vi "A33ConfigureFM.vi"(0 "VISA resource name":refnum<visa-resource-name>, 1 "Enable Frequency Modulation (T:Enable)":bool=TRUE, 2 "Modulation Frequency (1000.0 Hz)":dbl=1000.0 format="%#_12g", 5 "Channel (1: Channel1)":u16(ring)=1 items=["Channel1"=1, "Channel2"=2], 7 "FM Source (0: Internal)":u16(ring) items=["Internal", "External", "Channel 1", "Channel 2"], 9 "Modulation Waveform (0: Sine)":u16(ring) items=["Sine", "Square", "Triangle", "Ramp", "Negative Ramp", "Noise", "PRBS", "ARB"], 11 "error in (no error)":errorcluster, 13 "Modulation Deviation (100.0 Hz)":dbl=100.0 format="%#_12g") -> (4 "VISA resource name out":refnum<visa-resource-name>, 15 "error out":errorcluster)   [LabVIEW 2022 SP3]
doc: "Configures and enables amplitude modulation (AM). In AM, the amplitude of the carrier is varied by the amplitude of the modulating waveform. \n\n<B>Note:</B> The carrier waveform shape and parameters are set by the Configure Standard Waveform VI."
panel:
  # "Min 1uHz, Max 60 MHz"
  # "Min 1uHz to max for this WFM\nMax for TRIAG - 800 kHz"
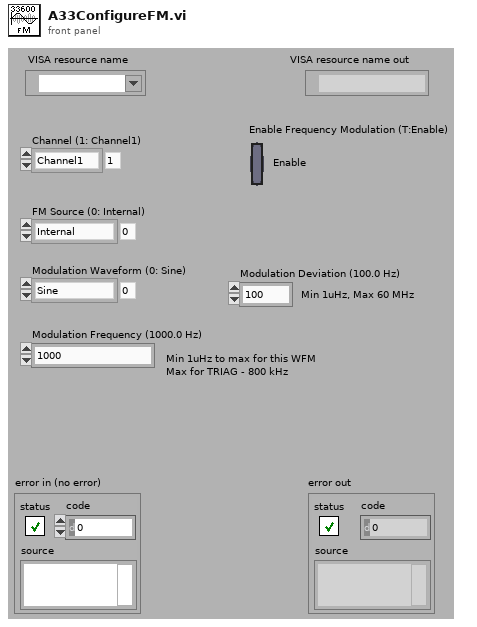
[diagram p1: front panel]
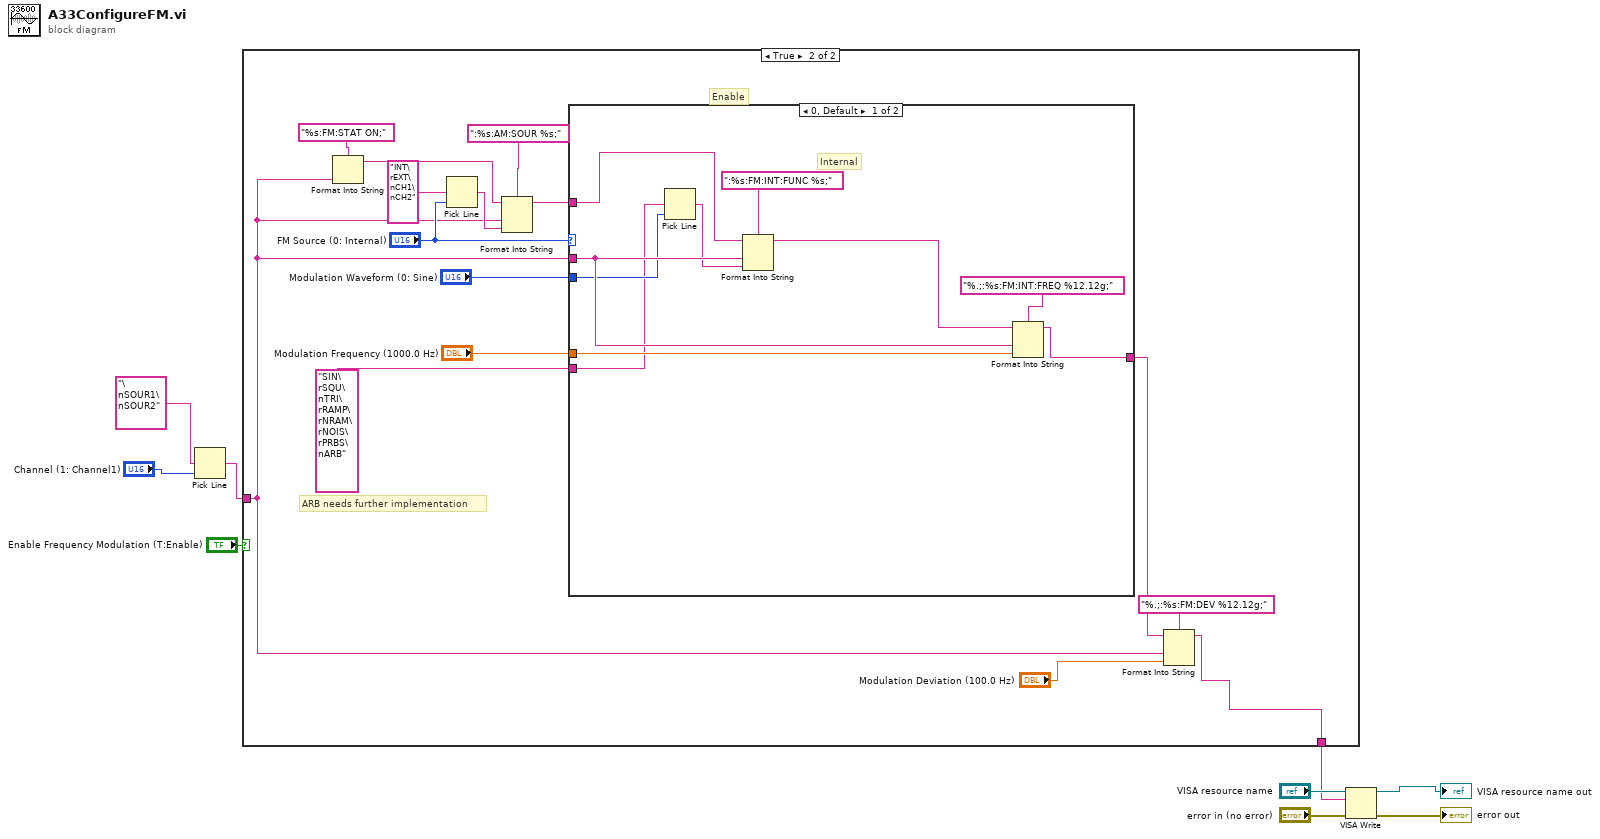
[diagram p0: block diagram]
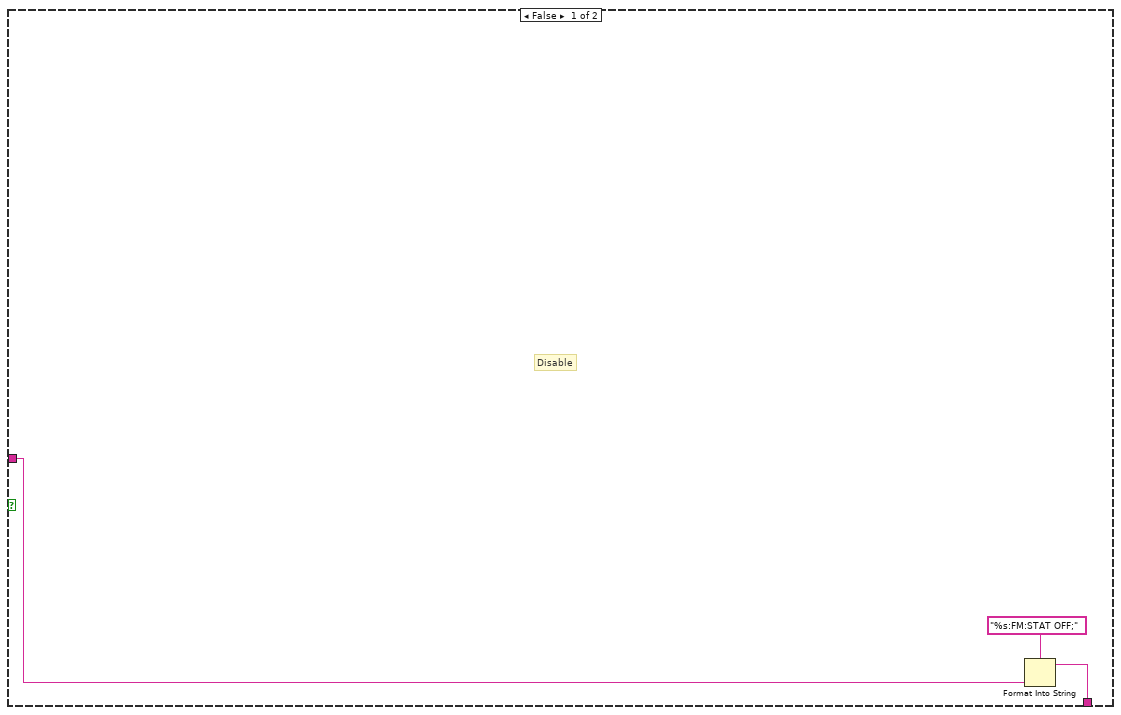
[diagram p2: hidden frame]
diagram:
  n1 = Pick Line(multi-line string="\nSOUR1\nSOUR2" ("string (\"\")"), line index="Channel (1: Channel1)") -> (output string=w1:string)  [unwired: 1 in]
  n2 = case shown="True" "Enable Frequency Modulation (T:Enable)" {
    tunnel: [w11 w13] -> w7
    tunnel: w1 -> [w10 w14]
    frame False {
      # "Disable"
      n3 = Format Into String(format string="%s:FM:STAT OFF;", w10) -> (resulting string=w11:string)  [unwired: 2 in, 1 out]
    }
    frame True {
      # "ARB needs further implementation"
      # "Enable"
      n4 = Format Into String(format string="%s:FM:STAT ON;", w14) -> (resulting string=w16:string)  [unwired: 2 in, 1 out]
      n5 = Pick Line(multi-line string="INT\rEXT\nCH1\nCH2", line index="FM Source (0: Internal)") -> (output string=w18:string)  [unwired: 1 in]
      n6 = Format Into String(format string=":%s:AM:SOUR %s;", initial string=w16, w14, w18) -> (resulting string=w20:string)  [unwired: 1 in, 1 out]
      n7 = case shown="0, Default" "FM Source (0: Internal)" {
        tunnel: w14 -> [w33 _]
        tunnel: [w35 w38] -> w26
        tunnel: "Modulation Waveform (0: Sine)" -> [w30 _]
        tunnel: "Modulation Frequency (1000.0 Hz)" -> [w34 _]
        tunnel: w20 -> [w31 w38]
        tunnel: "SIN\rSQU\nTRI\rRAMP\rNRAM\rNOIS\rPRBS\nARB" -> [w29 _]
        frame 0, Default {
          # "Internal"
          n8 = Pick Line(multi-line string=w29, line index=w30) -> (output string=w32:string)  [unwired: 1 in]
          n9 = Format Into String(format string=":%s:FM:INT:FUNC %s;", initial string=w31, w33, w32) -> (resulting string=w28:string)  [unwired: 1 in, 1 out]
          n10 = Format Into String(format string="%.;:%s:FM:INT:FREQ %12.12g;", initial string=w28, w33, w34) -> (resulting string=w35:string)  [unwired: 1 in, 1 out]
        }
        frame 1..3 {
          # "Other Channel or External"
        }
      }
      n11 = Format Into String(format string="%.;:%s:FM:DEV %12.12g;", initial string=w26, w14, "Modulation Deviation (100.0 Hz)") -> (resulting string=w13:string)  [unwired: 1 in, 1 out]
    }
  }
  n12 = VISA Write(VISA resource name="VISA resource name", write buffer=w7, error in (no error)="error in (no error)") -> (VISA resource name out=→"VISA resource name out":refnum<visa-resource-name>, error out=→"error out":errorcluster)  [unwired: 1 out]
